vi "Read.vi"(8 "error in (no error)":errorcluster, 11 "uCAN in":refnum<class "uCAN.lvclass">) -> (0 "error out":errorcluster, 1 "return count":u32, 2 "readout":string)   [LabVIEW 2021, in "uCanDriver.lvlib" / "uCAN.lvclass"]
uses:
  uCAN.lvclass
  uCAN.lvclass/uCAN.ctl
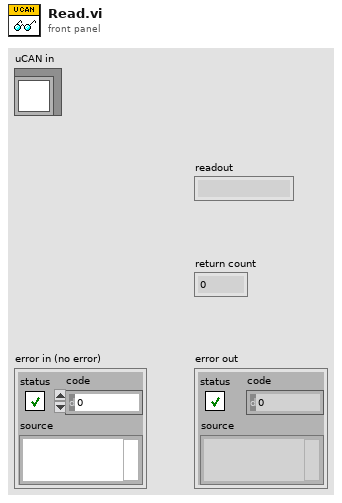
[diagram p1: front panel]
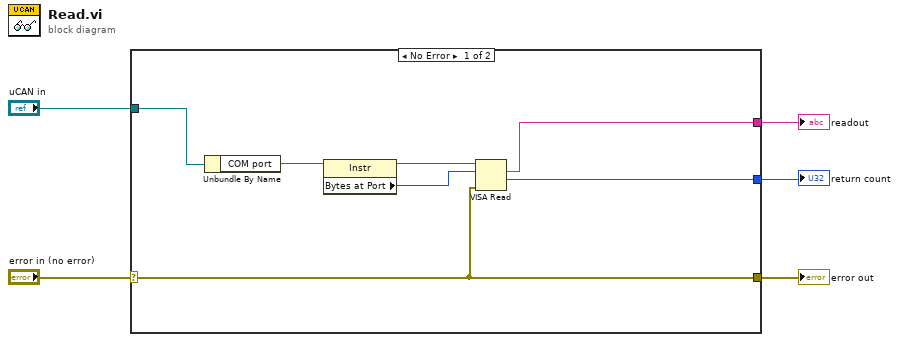
[diagram p0: block diagram]
diagram:
  n1 = case shown="No Error" "error in (no error)" {
    selector: "error in (no error)" -> [w8 w13]
    tunnel: [w8 w13] -> w4
    tunnel: "uCAN in" -> [w12 _]
    tunnel: [w7 _] -> w2
    tunnel: [w6 _] -> w1
    frame No Error {
      n2 = Unbundle By Name(w12) -> ("COM port"=w11:refnum<visa-resource-name>)
      n3 = property class="Instr"(reference=w11) -> (reference out=w10:refnum<visa-resource-name>, "Bytes at Port"=w9:u32)  [unwired: 1 in, 1 out]
      n4 = VISA Read(VISA resource name=w10, byte count=w9, error in (no error)=w8) -> (read buffer=w6:string, return count=w7:u32)  [unwired: 2 out]
    }
    frame Error {
    }
  }
  "error out" <- w4
  "return count" <- w2
  "readout" <- w1
